vi "poly_this_vis_path.vi"() -> (7 "your path":path)   [LabVIEW 2015]
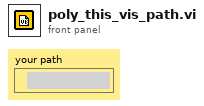
[diagram p1: front panel]
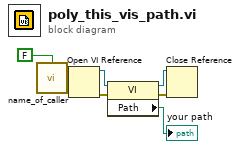
[diagram p0: block diagram]
diagram:
  n1 = call "name_of_caller.vi"("is in inlined vi? (F)"=FALSE) -> ("name of caller out"=w6:string)  [unwired: 3 in]
  n2 = Open VI Reference(vi path=w6) -> (vi reference=w5:refnum<vi>, error out=w3:errorcluster)  [unwired: 5 in]
  n3 = property class="VI"(reference=w5, error in=w3) -> (reference out=w4:refnum<vi>, error out=w2:errorcluster, "Path"=→"your path":path)
  n4 = Close Reference(reference=w4, error in (no error)=w2) -> ()  [unwired: 1 out]
